vi "Create Setter VI.vi"(8 "error in (no error)":errorcluster, 11 "Setter Generator In":refnum<class "Setter Generator.lvclass">) -> (0 "error out":errorcluster, 3 "Setter Generator Out":refnum<class "Setter Generator.lvclass">)   [LabVIEW 2020, in "Method Generation.lvlib" / "Setter Generator.lvclass"]
uses:
  Setter Generator.lvclass
  <vilib>/Utility/traverseref.llb/TRef TravTarget.ctl
  Setter Generator.lvclass/Setter Generator.ctl
  <vilib>/Utility/traverseref.llb/VI Scripting - Traverse.lvlib
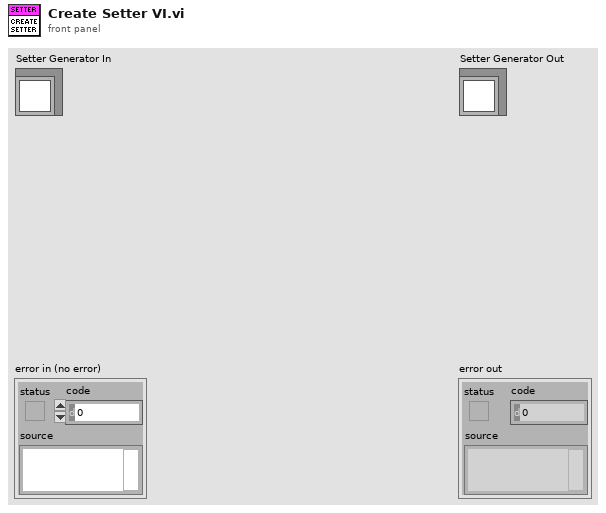
[diagram p1: front panel]
types:
  T1 = typedef "TRef TravTarget.ctl" = enum16{"FP", "BD", "Other"}
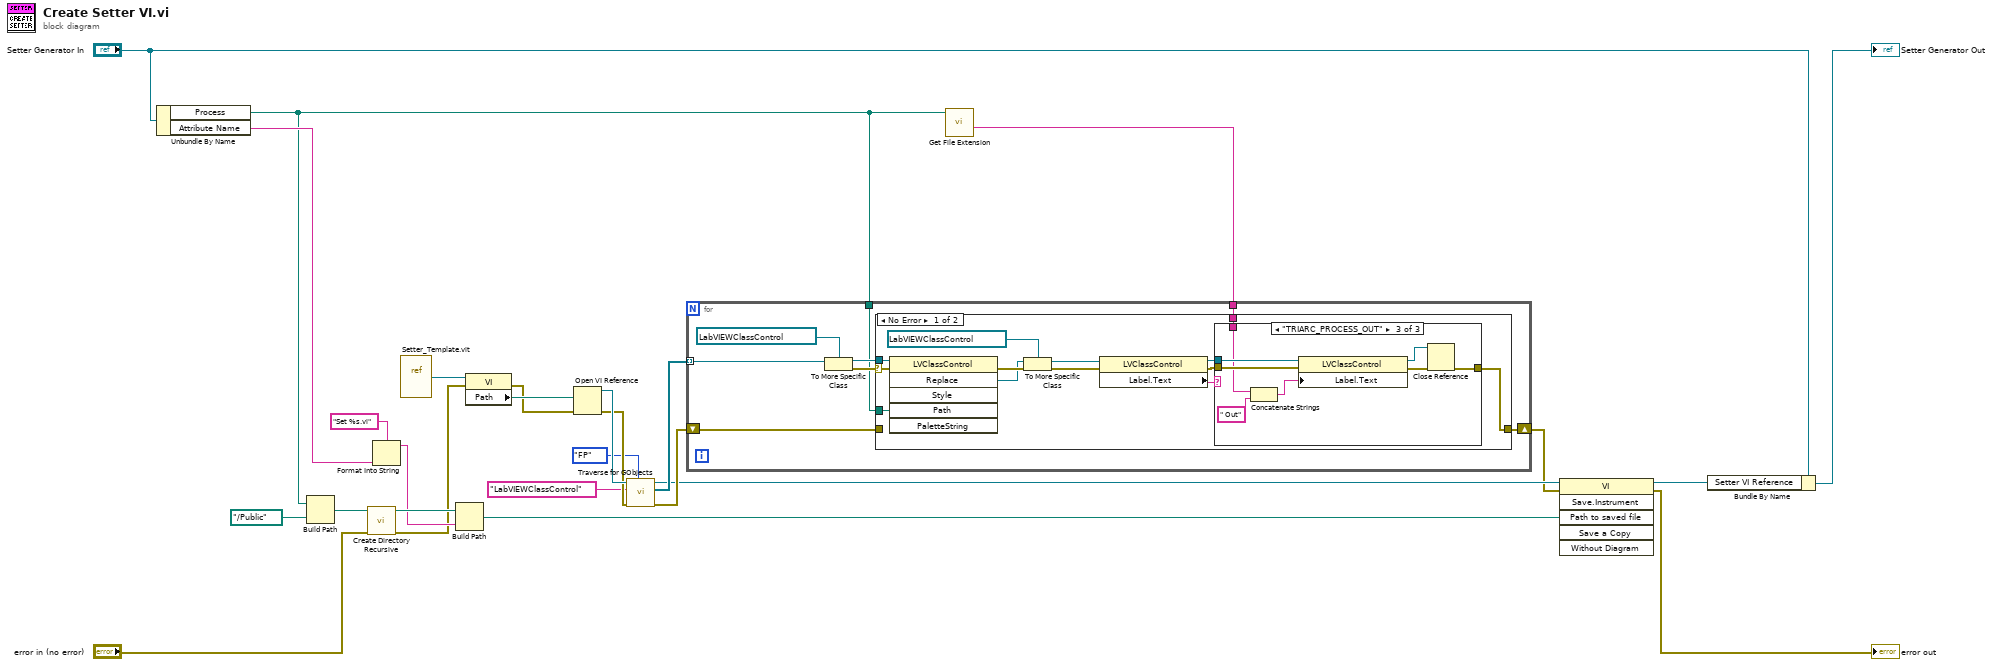
[diagram p0: block diagram]
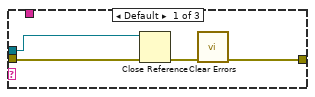
[diagram p2: hidden frame]
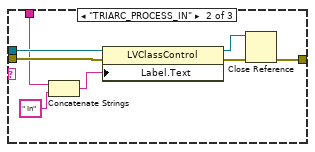
[diagram p3: hidden frame]
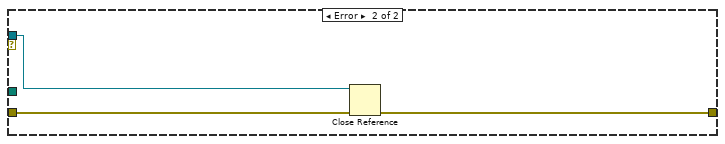
[diagram p4: hidden frame]
diagram:
  n1 = Unbundle By Name("Setter Generator In") -> ("Process"=w5:path, "Attribute Name"=w9:string)
  n2 = Build Path(base path=w5, name or relative path=path "../Public") -> (appended path=w14:path)
  n3 = call <vilib>:"Create Directory Recursive.vi"("error in (no error)"="error in (no error)", "directory"=w14) -> ("error out"=w7:errorcluster, "directory copy"=w11:path)  [unwired: 3 in, 1 out]
  n4 = Format Into String(format string="Set %s.vi", w9) -> (resulting string=w8:string)  [unwired: 2 in, 1 out]
  n5 = vi-ref "Setter_Template.vit"() -> (w26:refnum<vi>)
  n6 = Build Path(base path=w11, name or relative path=w8) -> (appended path=w12:path)
  n7 = property class="VI"(reference=w26, error in=w7) -> (error out=w22:errorcluster, "Path"=w23:path)  [unwired: 1 out]
  n8 = Open VI Reference(vi path=w23, error in (no error)=w22) -> (vi reference=w24:refnum<vi>, error out=w21:errorcluster)  [unwired: 4 in]
  n9 = call <vilib>:"Traverse for GObjects.vi"("Traverse Target"=TRef_TravTarget."FP", "error in (no error)"=w21, "Class Name"="LabVIEWClassControl", "VI Refnum"=w24) -> ("error out"=w18:errorcluster, "References"=w19:refnum<vi>[], "dup VI Refnum"=w16:refnum<vi>)  [unwired: 4 in, 1 out]
  n10 = call <vilib>:"Get File Extension.vi"("file"=w5) -> ("filename without extension"=w4:string)  [unwired: 6 in, 4 out]
  n11 = for {
    tunnel: w19 -> [w34] mode=indexing
    tunnel: w5 -> [w30]
    shift-right: [w29] -> w15
    shift-left: w18 -> [w28]
    tunnel: w4 -> [w27]
    n12 = To More Specific Class(target class=refnum<vi> refnum ("reference out"), reference=w34) -> (specific class reference=w31:refnum<vi>, error out=w32:errorcluster)  [unwired: 1 in]
    n13 = case shown="No Error" w32 {
      selector: w32 -> [w47 _]
      tunnel: w31 -> [w46 w68]
      tunnel: w30 -> [w45 _]
      tunnel: [w44 w69] -> w29
      tunnel: w28 -> [_ w70]
      tunnel: w27 -> [w41 _]
      frame No Error {
        n14 = invoke on="Invoke Node" class="LVClassControl" method="Replace"(reference=w46, error in=w47, "Path"=w45) -> (error out=w43:errorcluster, "Replace"=w38:refnum<vi>)  [unwired: 3 in, 4 out]
        n15 = To More Specific Class(target class=refnum<vi> refnum ("reference out"), reference=w38, error in=w43) -> (specific class reference=w37:refnum<vi>, error out=w36:errorcluster)
        n16 = property class="LVClassControl"(reference=w37, error in=w36) -> (reference out=w40:refnum<vi>, error out=w39:errorcluster, "Label.Text"=w42:string)
        n17 = case shown="\"TRIARC_PROCESS_OUT\"" w42 {
          tunnel: [w49 w53 w61] -> w44
          tunnel: w40 -> [w51 w58 w66]
          tunnel: w39 -> [w48 w57 w65]
          tunnel: w41 -> [_ w56 w64]
          frame Default {
            n18 = Close Reference(reference=w51, error in (no error)=w48) -> (error out=w50:errorcluster)
            n19 = call <vilib>:"Clear Errors.vi"("error in (no error)"=w50) -> ("error out"=w49:errorcluster)  [unwired: 5 in, 1 out]
          }
          frame "TRIARC_PROCESS_IN" {
            n20 = Concatenate Strings(w56, " In" ("string")) -> (w54:string)
            n21 = property class="LVClassControl"(reference=w58, error in=w57, "Label.Text"=w54) -> (reference out=w52:refnum<vi>, error out=w59:errorcluster)
            n22 = Close Reference(reference=w52, error in (no error)=w59) -> (error out=w53:errorcluster)
          }
          frame "TRIARC_PROCESS_OUT" {
            n23 = Concatenate Strings(w64, " Out" ("string")) -> (w62:string)
            n24 = property class="LVClassControl"(reference=w66, error in=w65, "Label.Text"=w62) -> (reference out=w60:refnum<vi>, error out=w67:errorcluster)
            n25 = Close Reference(reference=w60, error in (no error)=w67) -> (error out=w61:errorcluster)
          }
        }
      }
      frame Error {
        n26 = Close Reference(reference=w68, error in (no error)=w70) -> (error out=w69:errorcluster)
      }
    }
  }
  n27 = invoke on="Invoke Node" class="VI" method="Save.Instrument"(reference=w16, error in=w15, "Path to saved file"=w12) -> (reference out=w1:refnum<vi>, error out=→"error out":errorcluster)  [unwired: 3 in, 4 out]
  n28 = Bundle By Name(cluster="Setter Generator In", "Setter VI Reference"=w1) -> (→"Setter Generator Out":refnum<class "Setter Generator.lvclass">)
